vi "ProScan 3 Stage Engine.vi"(0 "Pro Scan 3 Notifier Name":string="ProScan3", 11 "COM Port":string[](array[string])) -> ()   [LabVIEW 2016]
uses:
  Stages Controls/Stage Notifier Element.ctl
  Stages Controls/Stage Actions.ctl
  Stages Controls/Stage Status.ctl
  <vilib>/Instr/_visa.llb/VISA Configure Serial Port (Instr).vi
panel:
  out "Backlash Status":string
  in  "Get Position":bool
  in  "XY Step Size (µm)":dbl format="%#_4g"
  in  "Y Position (µm)":dbl format="%#_4g"
  in  "X Position (µm)":dbl format="%#_4g"
  in  "Home":bool
  in  "Right":bool
  in  "Left":bool
  in  "Down":bool
  in  "Halt":bool
  in  "Up":bool
  in  "Quit":bool
  # "NOTE: Positions do not live update."
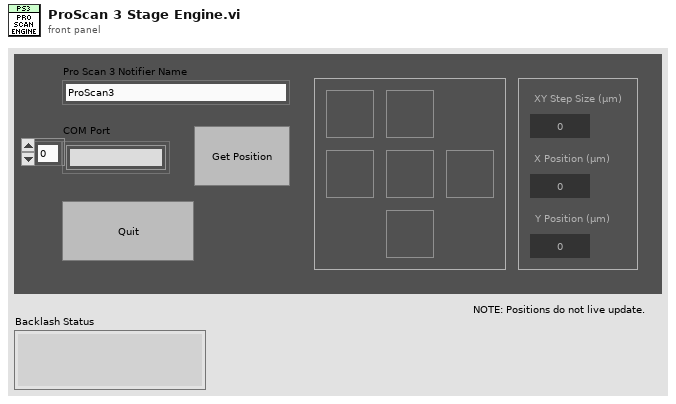
[diagram p1: front panel]
types:
  T1 = typedef "Stage Notifier Element.ctl" = cluster{"Action":T2, "Axis":bool[], "Setpoint":dbl[], "Velocity":dbl, "Cmd Recvd?":bool, "Position":dbl[], "Status":T3, "Misc":variant}
  T2 = typedef "Stage Actions.ctl" = enum16{"Get Position", "MVR", "MOVE", "HALT", "ONTARGET", "ERROR", "REFERENCE", "INIT", "VELOCITY", "STATUS", "EXIT", "HOME", "ZEROPOS", "NANOPOS", "ANALOG", "QUIT"}
  T3 = typedef "Stage Status.ctl" = enum16{"Error", "Abort", "Busy", "On Target"}
  T4 = enum32{"Invalid", "Standard", "Closed", "Hidden", "Minimized", "Maximized"}
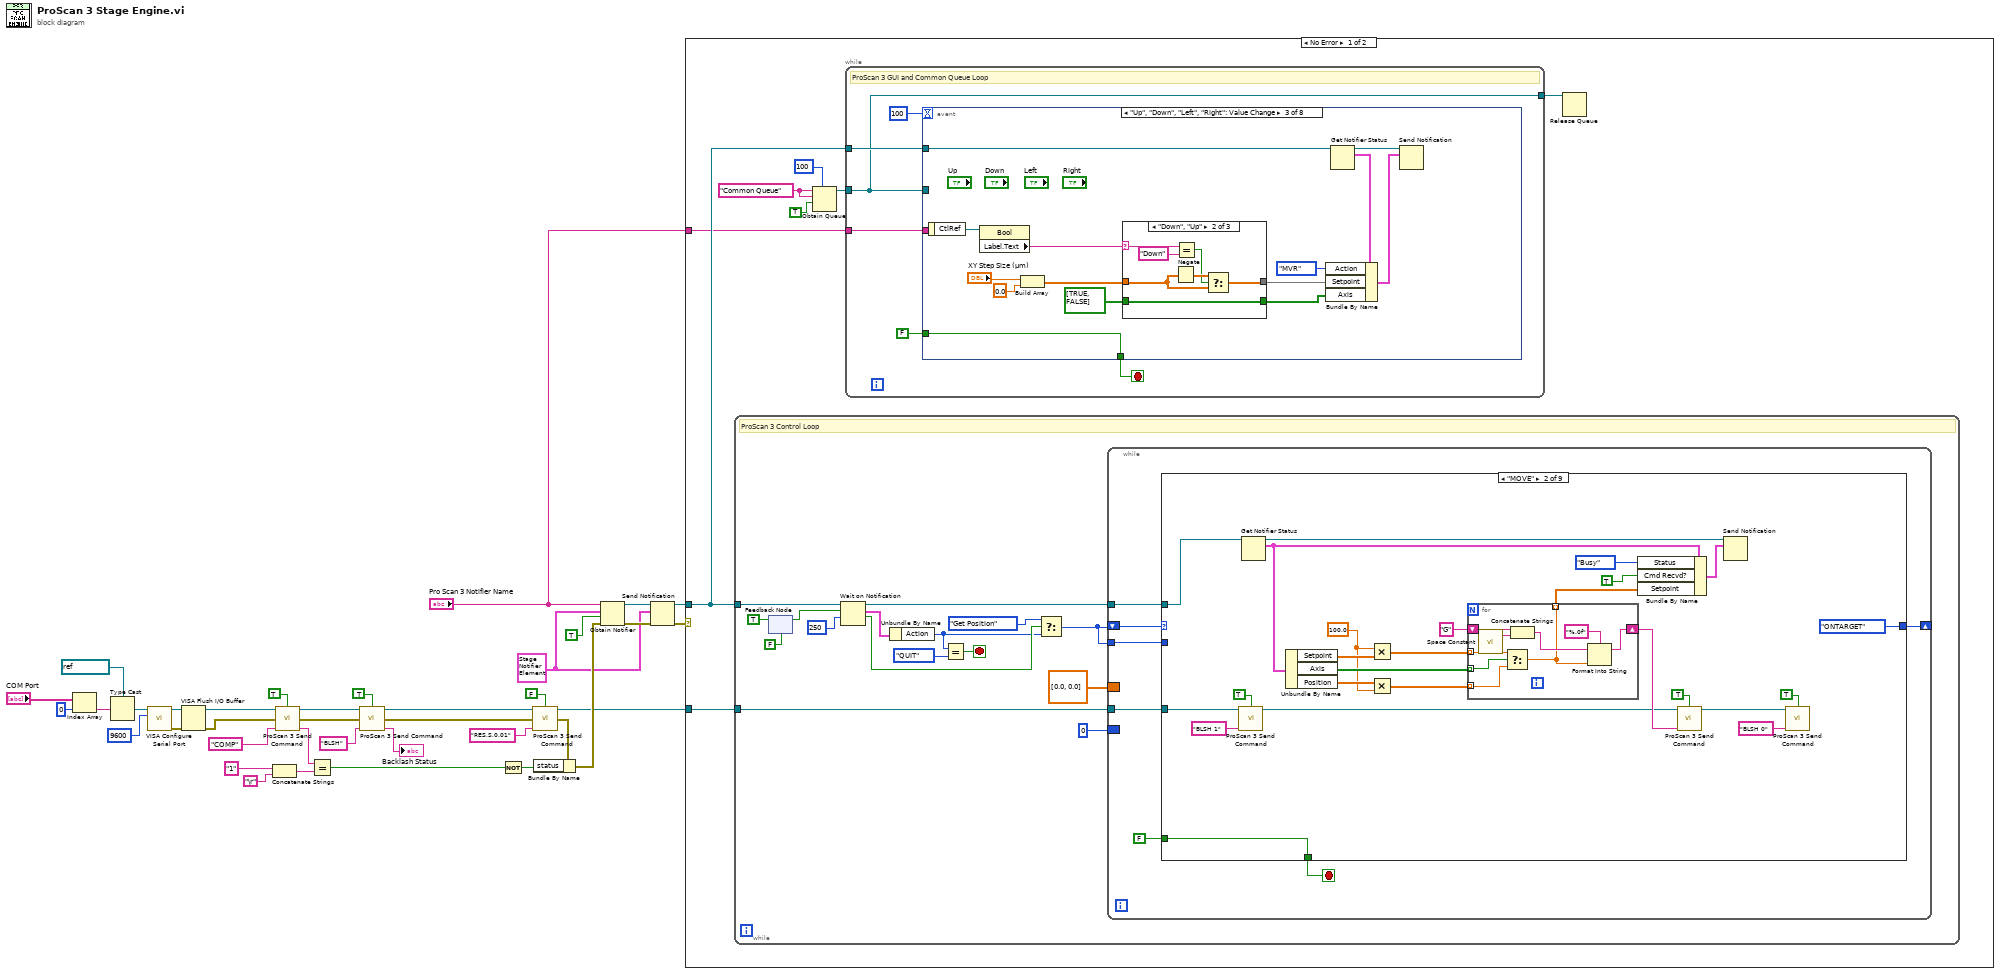
[diagram p0: block diagram]
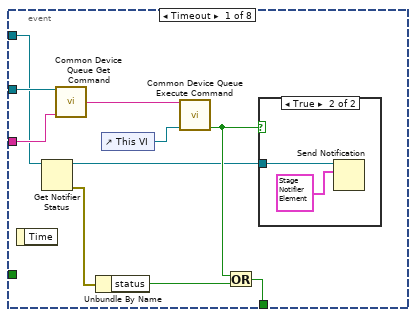
[diagram p2: hidden frame]
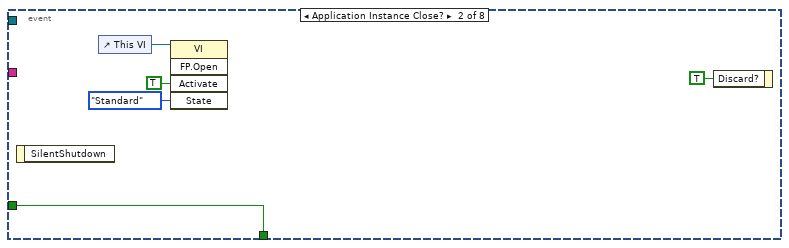
[diagram p4: hidden frame]
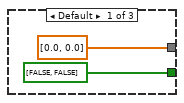
[diagram p5: hidden frame]
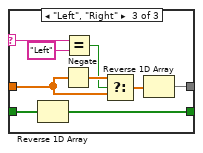
[diagram p6: hidden frame]
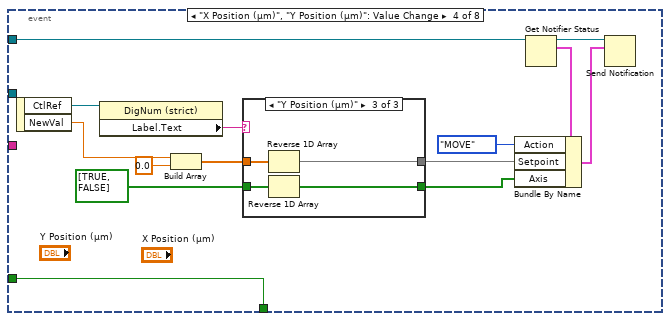
[diagram p7: hidden frame]
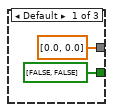
[diagram p8: hidden frame]
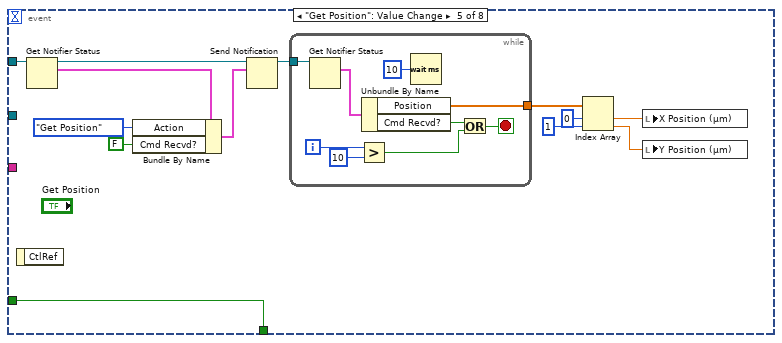
[diagram p10: hidden frame]
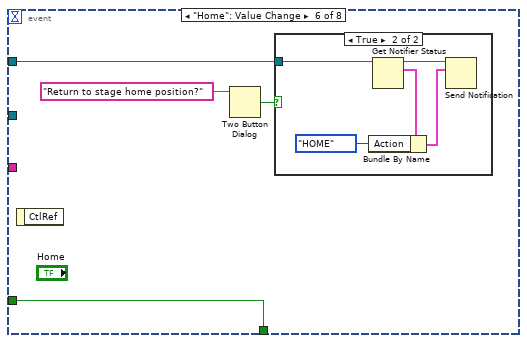
[diagram p11: hidden frame]
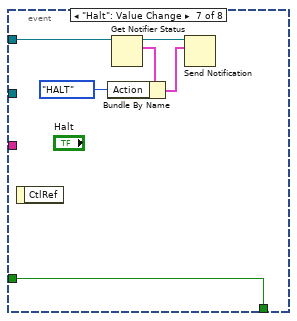
[diagram p13: hidden frame]
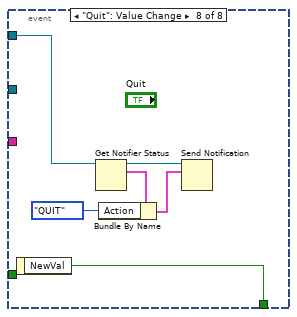
[diagram p14: hidden frame]
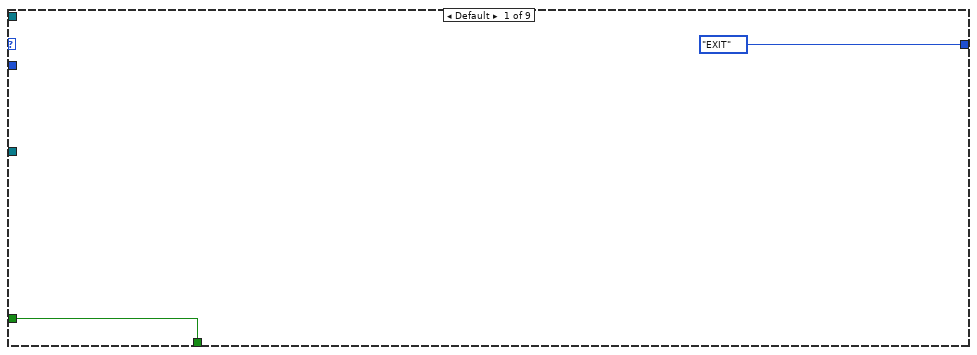
[diagram p15: hidden frame]
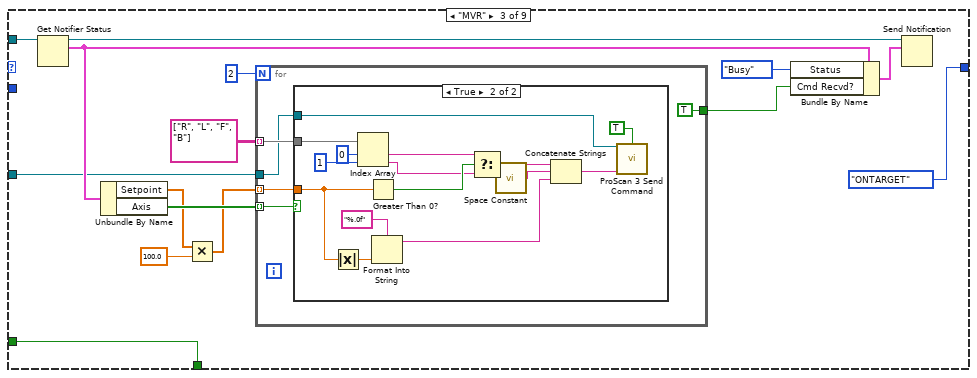
[diagram p16: hidden frame]
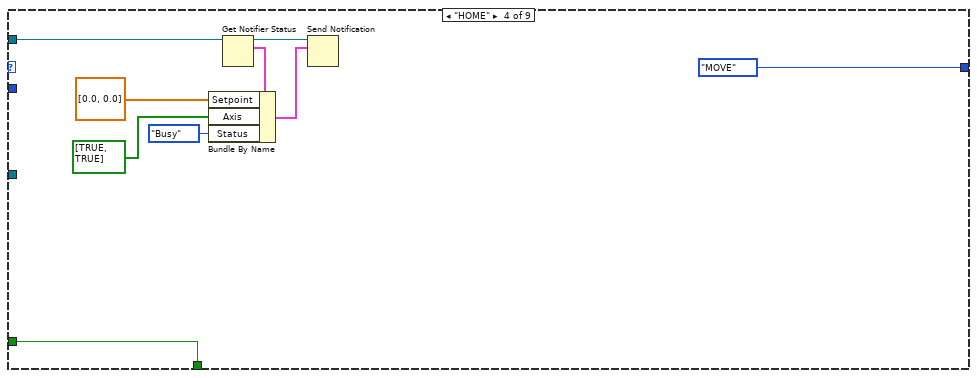
[diagram p18: hidden frame]
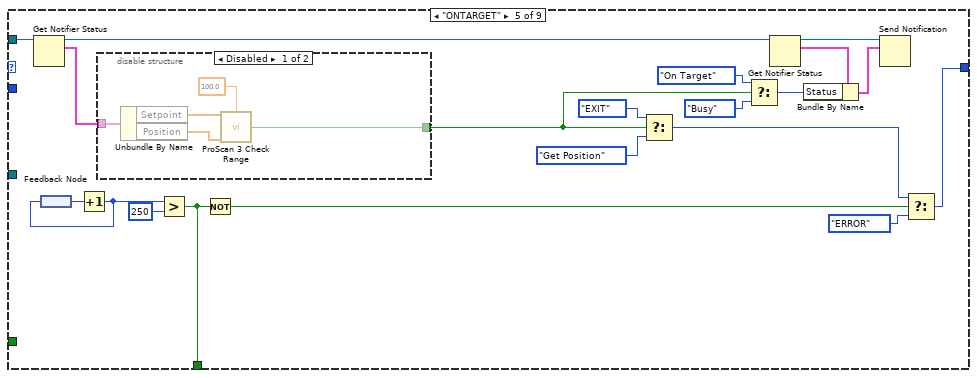
[diagram p19: hidden frame]
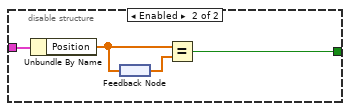
[diagram p20: hidden frame]
diagram:
  w19 = T1 {"Action"=enum."Get Position", "Axis"=[], "Setpoint"=[], "Velocity"=0.5, "Cmd Recvd?"=FALSE, "Position"=[], "Status"=enum."On Target", "Misc"=variant} ("Stage Status")
  n1 = Index Array(array="COM Port", index=0) -> (element=w15:string)
  n2 = Type Cast(type=refnum<visa-resource-name> "COM5" ("VISA resource name"), x=w15) -> (*(type *) &x=w14:refnum<visa-resource-name>)
  n3 = call-poly "VISA Configure Serial Port"("VISA resource name"=w14, "baud rate (9600)"=u32 9600) -> ("VISA resource name out"=w35:refnum<visa-resource-name>, "error out"=w34:errorcluster)  [unwired: 12 in]
  n4 = VISA Flush I/O Buffer(VISA resource name=w35, error in (no error)=w34) -> (VISA resource name out=w28:refnum<visa-resource-name>, error out=w27:errorcluster)  [unwired: 1 in]
  n5 = Concatenate Strings("1", "\r") -> (w31:string)
  n6 = call "ProScan 3 Send Command.vi"("VISA Ref"=w28, "Wait for Reply?"=TRUE, "Error In"=w27, "Command"="COMP") -> ("VISA Ref Out"=w5:refnum<visa-resource-name>, "Error Out"=w3:errorcluster, "Response"=w25:string)  [unwired: 9 in]
  n7 = Equal?(x=w25, y=w31) -> (x = y?=w30:bool)
  n8 = call "ProScan 3 Send Command.vi"("VISA Ref"=w5, "Wait for Reply?"=TRUE, "Error In"=w3, "Command"="BLSH") -> ("VISA Ref Out"=w4:refnum<visa-resource-name>, "Error Out"=w2:errorcluster, "Response"=→"Backlash Status":string)  [unwired: 9 in]
  n9 = Not(x=w30) -> (.not. x?=w29:bool)
  n10 = call "ProScan 3 Send Command.vi"("VISA Ref"=w4, "Wait for Reply?"=FALSE, "Error In"=w2, "Command"="RES,S,0.01") -> ("VISA Ref Out"=w11:refnum<visa-resource-name>, "Error Out"=w10:errorcluster)  [unwired: 9 in, 1 out]
  n11 = Bundle By Name(cluster=w10, "status"=w29) -> (w36:errorcluster)
  n12 = Obtain Notifier(name (unnamed)="Pro Scan 3 Notifier Name", notification data type=w19, create if not found? (T)=TRUE, error in (no error)=w36) -> (notifier out=w23:refnum<notifier>, error out=w22:errorcluster)  [unwired: 1 out]
  n13 = Send Notification(notification=w19, notifier=w23, error in (no error)=w22) -> (notifier out=w20:refnum<notifier>, error out=w21:errorcluster)
  n14 = case shown="No Error" w21 {
    selector: w21 -> [_ w408]
    tunnel: w20 -> [w41 w409]
    tunnel: w11 -> [w45 w410]
    tunnel: "Pro Scan 3 Notifier Name" -> [w40 _]
    frame No Error {
      w44 = "Common Queue" ("Unique Notifier Name")
      n15 = while {
        tunnel: w41 -> [w181]
        tunnel: w45 -> [w178]
        stop <- w177 stop-if-true
        # "ProScan 3 Control Loop"
        n16 = feedback-in #1(TRUE ("ignore previous (F)")) -> ()
        n17 = feedback #1(FALSE ("ignore previous (F)")) -> (w172:bool)
        n18 = Wait on Notification(notifier=w181, ignore previous (F)=w172, timeout in ms (-1)=250) -> (notifier out=w180:refnum<notifier>, notification=w176:T1, timed out?=w169:bool)  [unwired: 1 in, 1 out]
        n19 = Unbundle By Name(w176) -> ("Action"=w167:T2)
        n20 = Equal?(x=w167, y=Stage_Actions."QUIT") -> (x = y?=w177:bool)
        n21 = Select(t=Stage_Actions."Get Position", s=w169, f=w167) -> (s? t:f=w166:T2)
        n22 = while {
          tunnel: w180 -> [w188]
          tunnel: w178 -> [w186]
          shift-right: [w185] -> _
          shift-left: w166 -> [w187]
          tunnel: w166 -> [w182]
          border: 0 -> [_]
          border: dbl[] [0.0, 0.0] -> [_]
          stop <- w183 stop-if-true
          n23 = case shown="\"MOVE\"" w187 {
            selector: w187 -> [_ _ _ _ _ _ _ w362 _]
            tunnel: w188 -> [_ w211 w234 w264 w281 w319 w345 w364 w401]
            tunnel: w186 -> [_ w196 w229 _ _ w302 w350 w357 w399]
            tunnel: [Stage_Actions."EXIT" ("y") Stage_Actions."ONTARGET" ("y") Stage_Actions."ONTARGET" ("y") Stage_Actions."MOVE" ("y") w272 w304 w342 Stage_Actions."EXIT" ("y") Stage_Actions."QUIT" ("y")] -> w185
            tunnel: FALSE -> [w190 w215 w239 w262 _ w321 w338 _ _]
            tunnel: [w190 w215 w239 w262 w275 w321 w338 TRUE TRUE] -> w183
            tunnel: w182 -> [_ _ _ _ _ w303 _ _ _]
            frame Default {
            }
            frame "MOVE" {
              w200 = 100.0
              n24 = call "ProScan 3 Send Command.vi"("VISA Ref"=w196, "Wait for Reply?"=TRUE, "Command"="BLSH 1") -> ("VISA Ref Out"=w195:refnum<visa-resource-name>)  [unwired: 10 in, 2 out]
              n25 = Get Notifier Status(notifier=w211) -> (notifier out=w213:refnum<notifier>, current notification=w206:T1)  [unwired: 1 in, 3 out]
              n26 = Unbundle By Name(w206) -> ("Setpoint"=w202:dbl[], "Axis"=w207:bool[], "Position"=w201:dbl[])
              n27 = Multiply(x=w200, y=w202) -> (x*y=w198:dbl[])
              n28 = Multiply(x=w201, y=w200) -> (x*y=w199:dbl[])
              n29 = for {
                tunnel: w207 -> [w223] mode=indexing
                tunnel: w199 -> [w217] mode=indexing
                tunnel: w198 -> [w224] mode=indexing
                shift-right: [w218] -> w203
                shift-left: "G" ("f") -> [w221]
                tunnel: [w216] -> w204 mode=indexing
                n30 = call <vilib>:"Space Constant.vi"() -> ("String"=w220:string)
                n31 = Select(t=w224, s=w223, f=w217) -> (s? t:f=w216:dbl)
                n32 = Concatenate Strings(w221, w220) -> (w219:string)
                n33 = Format Into String(format string="%.0f", initial string=w219, w216) -> (resulting string=w218:string)  [unwired: 1 in, 1 out]
              }
              n34 = Bundle By Name(cluster=w206, "Status"=Stage_Status."Busy", "Cmd Recvd?"=TRUE, "Setpoint"=w204) -> (w212:T1)
              n35 = call "ProScan 3 Send Command.vi"("VISA Ref"=w195, "Wait for Reply?"=TRUE, "Command"=w203) -> ("VISA Ref Out"=w191:refnum<visa-resource-name>)  [unwired: 10 in, 2 out]
              n36 = Send Notification(notification=w212, notifier=w213) -> ()  [unwired: 1 in, 2 out]
              n37 = call "ProScan 3 Send Command.vi"("VISA Ref"=w191, "Wait for Reply?"=TRUE, "Command"="BLSH 0") -> ()  [unwired: 10 in, 3 out]
            }
            frame "MVR" {
              n38 = Get Notifier Status(notifier=w234) -> (notifier out=w236:refnum<notifier>, current notification=w233:T1)  [unwired: 1 in, 3 out]
              n39 = Unbundle By Name(w233) -> ("Setpoint"=w227:dbl[], "Axis"=w232:bool[])
              n40 = Multiply(x=w227, y=100.0) -> (x*y=w225:dbl[])
              n41 = for {
                N: 2 -> [_]
                tunnel: w232 -> [w244] mode=indexing
                tunnel: w225 -> [w243] mode=indexing
                tunnel: string[][] [["R", "L"], ["F", "B"]] -> [w242] mode=indexing
                tunnel: w229 -> [w241]
                tunnel: [TRUE ("Cmd Recvd?")] -> w228
                n42 = case shown="True" w244 {
                  tunnel: w243 -> [_ w252]
                  tunnel: w242 -> [_ w259]
                  tunnel: w241 -> [_ w245]
                  frame False {
                  }
                  frame True {
                    n43 = Absolute Value(x=w252) -> (abs(x)=w248:dbl)
                    n44 = Index Array(array=w259, index #1=0 ("index"), index #2=1 ("index")) -> (element #1=w254:string, element #2=w255:string)
                    n45 = Greater Than 0?(x=w252) -> (x > 0?=w256:bool)
                    n46 = Format Into String(format string="%.0f", w248) -> (resulting string=w249:string)  [unwired: 2 in, 1 out]
                    n47 = Select(t=w254, s=w256, f=w255) -> (s? t:f=w251:string)
                    n48 = call <vilib>:"Space Constant.vi"() -> ("String"=w250:string)
                    n49 = Concatenate Strings(w251, w250, w249) -> (w246:string)
                    n50 = call "ProScan 3 Send Command.vi"("VISA Ref"=w245, "Wait for Reply?"=TRUE, "Command"=w246) -> ()  [unwired: 10 in, 3 out]
                  }
                }
              }
              n51 = Bundle By Name(cluster=w233, "Status"=Stage_Status."Busy", "Cmd Recvd?"=w228) -> (w235:T1)
              n52 = Send Notification(notification=w235, notifier=w236) -> ()  [unwired: 1 in, 2 out]
            }
            frame "HOME" {
              n53 = Get Notifier Status(notifier=w264) -> (notifier out=w266:refnum<notifier>, current notification=w267:T1)  [unwired: 1 in, 3 out]
              n54 = Bundle By Name(cluster=w267, "Setpoint"=dbl[] [0.0, 0.0], "Axis"=bool[] [TRUE, TRUE], "Status"=Stage_Status."Busy") -> (w265:T1)
              n55 = Send Notification(notification=w265, notifier=w266) -> ()  [unwired: 1 in, 2 out]
            }
            frame "ONTARGET" {
              n56 = Get Notifier Status(notifier=w281) -> (notifier out=w280:refnum<notifier>, current notification=w279:T1)  [unwired: 1 in, 3 out]
              n57 = feedback #2() -> (w278:i32)
              n58 = Increment(x=w278) -> (x+1=w277:i32)
              n59 = feedback-in #2(w277) -> ()
              n60 = disable-structure shown="Disabled" {
                disable-tunnel: w279 -> [w293 w297]
                disable-tunnel: [w289 w294] -> w269
                frame Disabled {
                  n61 = Unbundle By Name(w293) -> ("Setpoint"=w292:dbl[], "Position"=w291:dbl[])
                  n62 = call "ProScan 3 Check Range.vi"("Setpoint"=w292, "Range Limit"=100.0, "Position"=w291) -> ("In Range?"=w289:bool)  [unwired: 12 in]
                }
                frame Enabled {
                  n63 = Unbundle By Name(w297) -> ("Position"=w295:dbl[])
                  n64 = feedback-in #3(w295) -> ()
                  n65 = feedback #3() -> (w296:dbl[])
                  n66 = Equal?(x=w295, y=w296) -> (x = y?=w294:bool)
                }
              }
              n67 = Greater?(x=w277, y=250) -> (0:w275:bool)
              n68 = Not(x=w275) -> (.not. x?=w271:bool)
              n69 = Select(t=Stage_Actions."EXIT" ("y"), s=w269, f=Stage_Actions."Get Position" ("y")) -> (s? t:f=w274:T2)
              n70 = Select(t=Stage_Status."On Target" ("Status"), s=w269, f=Stage_Status."Busy" ("Status")) -> (s? t:f=w282:T3)
              n71 = Get Notifier Status(notifier=w280) -> (notifier out=w286:refnum<notifier>, current notification=w287:T1)  [unwired: 1 in, 3 out]
              n72 = Bundle By Name(cluster=w287, "Status"=w282) -> (w285:T1)
              n73 = Send Notification(notification=w285, notifier=w286) -> ()  [unwired: 1 in, 2 out]
              n74 = Select(t=w274, s=w271, f=Stage_Actions."ERROR") -> (s? t:f=w272:T2)
            }
            frame "Get Position" {
              w312 = "," ("regular expression")
              n75 = VISA Flush I/O Buffer(VISA resource name=w302) -> (VISA resource name out=w301:refnum<visa-resource-name>)  [unwired: 2 in, 1 out]
              n76 = call "ProScan 3 Send Command.vi"("VISA Ref"=w301, "Wait for Reply?"=TRUE, "Command"="P") -> ("Response"=w307:string)  [unwired: 10 in, 2 out]
              n77 = Search and Replace String(input string=w307, search string="[a-zA-Z]", replace string="") -> (result string=w310:string)  [unwired: 5 in, 3 out]
              n78 = Match Pattern(string=w310, regular expression=w312) -> (before substring=w313:string, after substring=w311:string)  [unwired: 1 in, 2 out]
              n79 = Match Pattern(string=w311, regular expression=w312) -> (before substring=w314:string, after substring=w315:string)  [unwired: 1 in, 2 out]
              n80 = Build Array(w313, w314, w315) -> (w316:string[])
              n81 = for {
                N: 2 -> [_]
                tunnel: w316 -> [w335] mode=indexing
                tunnel: [w333] -> w300 mode=indexing
                n82 = call <vilib>:"Trim Whitespace.vi"("string"=w335) -> ("trimmed string"=w332:string)  [unwired: 1 in]
                n83 = Decimal String To Number(string=w332, default (0L)=0.0) -> (number=w333:dbl)  [unwired: 1 in, 1 out]
              }
              n84 = Divide(x=w300, y=100.0) -> (x/y=w298:dbl[])
              n85 = Get Notifier Status(notifier=w319) -> (notifier out=w322:refnum<notifier>, current notification=w306:T1)  [unwired: 1 in, 3 out]
              n86 = case shown="Default" w303 {
                tunnel: w306 -> [w326 w331]
                tunnel: [w325 w330] -> w305
                tunnel: w298 -> [w324 w329]
                tunnel: [Stage_Actions."ONTARGET" ("y") Stage_Actions."EXIT" ("y")] -> w304
                frame Default {
                  n87 = Bundle By Name(cluster=w326, "Position"=w324) -> (w325:T1)
                }
                frame "Get Position", "HALT" {
                  n88 = Bundle By Name(cluster=w331, "Position"=w329, "Cmd Recvd?"=TRUE) -> (w330:T1)
                }
              }
              n89 = Send Notification(notification=w305, notifier=w322) -> ()  [unwired: 1 in, 2 out]
            }
            frame "HALT" {
              n90 = call "ProScan 3 Send Command.vi"("VISA Ref"=w350, "Wait for Reply?"=TRUE, "Command"="I" ("string")) -> ("Response"=w351:string)  [unwired: 10 in, 2 out]
              n91 = Concatenate Strings("R" ("y"), "\r") -> (w353:string)
              n92 = Equal?(x=w351, y=w353) -> (x = y?=w341:bool)
              n93 = Select(t=Stage_Status."Abort" ("Status"), s=w341, f=Stage_Status."Error" ("Status")) -> (s? t:f=w337:T3)
              n94 = Select(t=Stage_Actions."Get Position" ("y"), s=w341, f=Stage_Actions."ERROR" ("y")) -> (s? t:f=w342:T2)
              n95 = Get Notifier Status(notifier=w345) -> (notifier out=w348:refnum<notifier>, current notification=w349:T1)  [unwired: 1 in, 3 out]
              n96 = Bundle By Name(cluster=w349, "Status"=w337, "Cmd Recvd?"=TRUE) -> (w347:T1)
              n97 = Send Notification(notification=w347, notifier=w348) -> ()  [unwired: 1 in, 2 out]
            }
            frame "ERROR".."EXIT" {
              n98 = case shown="Default" w362 {
                tunnel: w364 -> [w390 w396]
                tunnel: [w390 w391] -> w356
                frame Default {
                }
                frame "ERROR" {
                  n99 = Get Notifier Status(notifier=w396) -> (notifier out=w393:refnum<notifier>, current notification=w395:T1)  [unwired: 1 in, 3 out]
                  n100 = Bundle By Name(cluster=w395, "Status"=Stage_Status."Error") -> (w392:T1)
                  n101 = Send Notification(notification=w392, notifier=w393) -> (notifier out=w391:refnum<notifier>)  [unwired: 1 in, 1 out]
                }
              }
              n102 = Get Notifier Status(notifier=w356) -> (notifier out=w360:refnum<notifier>, current notification=w359:T1)  [unwired: 1 in, 3 out]
              n103 = disable-structure shown="Enabled" {
                disable-tunnel: w359 -> [w371 w389]
                disable-tunnel: [w370 w389] -> w358
                disable-tunnel: w357 -> [w365 _]
                frame Disabled {
                  w377 = "," ("regular expression")
                  n104 = VISA Flush I/O Buffer(VISA resource name=w365) -> (VISA resource name out=w369:refnum<visa-resource-name>)  [unwired: 2 in, 1 out]
                  n105 = call "ProScan 3 Send Command.vi"("VISA Ref"=w369, "Wait for Reply?"=TRUE, "Command"="P") -> ("Response"=w372:string)  [unwired: 10 in, 2 out]
                  n106 = Search and Replace String(input string=w372, search string="[a-zA-Z]", replace string="") -> (result string=w375:string)  [unwired: 5 in, 3 out]
                  n107 = Match Pattern(string=w375, regular expression=w377) -> (before substring=w378:string, after substring=w376:string)  [unwired: 1 in, 2 out]
                  n108 = Match Pattern(string=w376, regular expression=w377) -> (before substring=w379:string, after substring=w380:string)  [unwired: 1 in, 2 out]
                  n109 = Build Array(w378, w379, w380) -> (w381:string[])
                  n110 = for {
                    N: 2 -> [_]
                    tunnel: w381 -> [w388] mode=indexing
                    tunnel: [w386] -> w368 mode=indexing
                    n111 = call <vilib>:"Trim Whitespace.vi"("string"=w388) -> ("trimmed string"=w385:string)  [unwired: 1 in]
                    n112 = Decimal String To Number(string=w385, default (0L)=0.0) -> (number=w386:dbl)  [unwired: 1 in, 1 out]
                  }
                  n113 = Divide(x=w368, y=100.0) -> (x/y=w366:dbl[])
                  n114 = Bundle By Name(cluster=w371, "Position"=w366) -> (w370:T1)
                }
                frame Enabled {
                }
              }
              n115 = Send Notification(notification=w358, notifier=w360) -> ()  [unwired: 1 in, 2 out]
            }
            frame "QUIT" {
              n116 = Release Notifier(notifier=w401, force destroy? (F)=TRUE) -> ()  [unwired: 1 in, 3 out]
              n117 = VISA Close(VISA resource name=w399) -> ()  [unwired: 1 in, 1 out]
            }
          }
        }
      }
      n118 = Obtain Queue(max queue size (-1, unlimited)=100, name (unnamed)=w44, element data type=w44, create if not found? (T)=TRUE) -> (queue out=w42:refnum<queue>)  [unwired: 1 in, 2 out]
      n119 = while {
        tunnel: w42 -> [w46]
        tunnel: w40 -> [w49]
        tunnel: w41 -> [w50]
        tunnel: [w46] -> w38
        stop <- w48 stop-if-true
        # "ProScan 3 GUI and Common Queue Loop"
        n120 = event shown="[2] \"Up\", \"Down\", \"Left\", \"Right\": Value Change" {
          selector: _ -> [_ _ _ _ _ _ _ _]
          dyn-events: _ -> [_ _ _ _ _ _ _ _]
          timeout: 100 -> [_ _ _ _ _ _ _ _]
          tunnel: w46 -> [w55 _ _ _ _ _ _ _]
          tunnel: w50 -> [w52 _ w75 w107 w134 w145 w158 w165]
          tunnel: w49 -> [w54 _ _ _ _ _ _ _]
          tunnel: [w53 w68 w78 w114 w135 w147 w159 w161] -> w48
          tunnel: FALSE -> [_ w68 w78 w114 w135 w147 w159 _]
          event Timeout {
            n121 = event-data() -> ()  [unwired: 1 in, 1 out]
            n122 = Get Notifier Status(notifier=w52) -> (notifier out=w56:refnum<notifier>, error out=w61:errorcluster)  [unwired: 1 in, 3 out]
            n123 = call "Common Device Queue Get Command.vi"("Common Queue"=w55, "Notifier Name"=w54) -> ("Command"=w60:string)  [unwired: 12 in, 1 out]
            n124 = Unbundle By Name(w61) -> ("status"=w58:bool)
            n125 = control-ref of="This VI"() -> (w59:refnum<vi>)
            n126 = call "Common Device Queue Execute Command.vi"("Common Command"=w60, "VI Refnum"=w59) -> ("Quit?"=w57:bool)  [unwired: 12 in, 1 out]
            n127 = Or(x=w57, y=w58) -> (x .or. y?=w53:bool)
            n128 = case shown="True" w57 {
              tunnel: w56 -> [_ w63]
              frame False {
              }
              frame True {
                n129 = Send Notification(notification=T1 {"Action"=enum."QUIT", "Axis"=[], "Setpoint"=[], "Velocity"=0.5, "Cmd Recvd?"=FALSE, "Position"=[], "Status"=enum."Error", "Misc"=variant} ("Stage Status"), notifier=w63) -> ()  [unwired: 1 in, 2 out]
              }
            }
          }
          event Application Instance Close? {
            n130 = event-data() -> ()  [unwired: 1 in, 1 out]
            n131 = control-ref of="This VI"() -> (w65:refnum<vi>)
            n132 = invoke class="VI" method="FP.Open"(reference=w65, "Activate"=TRUE ("Activate?"), "State"=T4."Standard") -> ()  [unwired: 2 in, 5 out]
            n133 = event-data("Discard?"=TRUE) -> ()  [unwired: 1 in, 1 out]
          }
          event "Up", "Down", "Left", "Right": Value Change {
            n134 = event-data() -> ("CtlRef"=w77:refnum<vi>)  [unwired: 1 in]
            n135 = property class="Bool"(reference=w77) -> ("Label.Text"=w82:string)  [unwired: 1 in, 2 out]
            n136 = Build Array("XY Step Size (µm)", 0.0 ("element")) -> (w80:dbl[])
            n137 = case shown="\"Down\", \"Up\"" w82 {
              selector: w82 -> [_ w91 w97]
              tunnel: w80 -> [_ w88 w96]
              tunnel: bool[] [TRUE, FALSE] -> [_ w85 w94]
              tunnel: [dbl[] [0.0, 0.0] w87 w93] -> w73
              tunnel: [bool[] [FALSE, FALSE] w85 w92] -> w72
              frame Default {
              }
              frame "Down", "Up" {
                n138 = Negate(x=w88) -> (-x=w89:dbl[])
                n139 = Equal?(x=w91, y="Down") -> (x = y?=w86:bool)
                n140 = Select(t=w89, s=w86, f=w88) -> (s? t:f=w87:dbl[])
              }
              frame "Left", "Right" {
                n141 = Reverse 1D Array(array=w94) -> (reversed array=w92:bool[])
                n142 = Negate(x=w96) -> (-x=w99:dbl[])
                n143 = Equal?(x=w97, y="Left") -> (x = y?=w98:bool)
                n144 = Select(t=w99, s=w98, f=w96) -> (s? t:f=w95:dbl[])
                n145 = Reverse 1D Array(array=w95) -> (reversed array=w93:dbl[])
              }
            }
            n146 = Get Notifier Status(notifier=w75) -> (notifier out=w70:refnum<notifier>, current notification=w74:T1)  [unwired: 1 in, 3 out]
            n147 = Bundle By Name(cluster=w74, "Action"=Stage_Actions."MVR", "Setpoint"=w73, "Axis"=w72) -> (w69:T1)
            n148 = Send Notification(notification=w69, notifier=w70) -> ()  [unwired: 1 in, 2 out]
          }
          event "X Position (µm)", "Y Position (µm)": Value Change {
            n149 = event-data() -> ("CtlRef"=w109:refnum<vi>, "NewVal"=w108:dbl)  [unwired: 1 in]
            n150 = property class="DigNum (strict)"(reference=w109) -> ("Label.Text"=w112:string)  [unwired: 1 in, 2 out]
            n151 = Build Array(w108, 0.0 ("element")) -> (w113:dbl[])
            n152 = case shown="\"Y Position (µm)\"" w112 {
              tunnel: w113 -> [_ w118 w122]
              tunnel: bool[] [TRUE, FALSE] -> [_ w117 w121]
              tunnel: [dbl[] [0.0, 0.0] w118 w120] -> w104
              tunnel: [bool[] [FALSE, FALSE] w117 w119] -> w103
              frame Default {
              }
              frame "X Position (µm)" {
              }
              frame "Y Position (µm)" {
                n153 = Reverse 1D Array(array=w122) -> (reversed array=w120:dbl[])
                n154 = Reverse 1D Array(array=w121) -> (reversed array=w119:bool[])
              }
            }
            n155 = Get Notifier Status(notifier=w107) -> (notifier out=w106:refnum<notifier>, current notification=w105:T1)  [unwired: 1 in, 3 out]
            n156 = Bundle By Name(cluster=w105, "Action"=Stage_Actions."MOVE", "Setpoint"=w104, "Axis"=w103) -> (w101:T1)
            n157 = Send Notification(notification=w101, notifier=w106) -> ()  [unwired: 1 in, 2 out]
          }
          event "Get Position": Value Change {
            n158 = event-data() -> ()  [unwired: 1 in, 1 out]
            n159 = Get Notifier Status(notifier=w134) -> (notifier out=w133:refnum<notifier>, current notification=w132:T1)  [unwired: 1 in, 3 out]
            n160 = Bundle By Name(cluster=w132, "Action"=Stage_Actions."Get Position", "Cmd Recvd?"=FALSE) -> (w129:T1)
            n161 = Send Notification(notification=w129, notifier=w133) -> (notifier out=w128:refnum<notifier>)  [unwired: 1 in, 1 out]
            n162 = while {
              tunnel: w128 -> [w144]
              tunnel: [w136] -> w127
              i -> [w140]
              stop <- w137 stop-if-true
              n163 = Get Notifier Status(notifier=w144) -> (current notification=w143:T1)  [unwired: 1 in, 4 out]
              n164 = Greater?(x=w140, y=10) -> (0:w138:bool)
              n165 = Unbundle By Name(w143) -> ("Position"=w136:dbl[], "Cmd Recvd?"=w139:bool)
              n166 = Wait (ms)(milliseconds to wait=u32 10) -> ()  [unwired: 1 out]
              n167 = Or(x=w139, y=w138) -> (x .or. y?=w137:bool)
            }
            n168 = Index Array(array=w127, index #1=0 ("index"), index #2=1 ("index")) -> (element #1=w124:dbl, element #2=w123:dbl)
            n169 = local write "X Position (µm)"(w124) -> ()
            n170 = local write "Y Position (µm)"(w123) -> ()
          }
          event "Home": Value Change {
            n171 = event-data() -> ()  [unwired: 1 in, 1 out]
            n172 = Two Button Dialog(message="Return to stage home position?") -> (T button?=w146:bool)  [unwired: 2 in]
            n173 = case shown="True" w146 {
              tunnel: w145 -> [_ w153]
              frame False {
              }
              frame True {
                n174 = Get Notifier Status(notifier=w153) -> (notifier out=w152:refnum<notifier>, current notification=w151:T1)  [unwired: 1 in, 3 out]
                n175 = Bundle By Name(cluster=w151, "Action"=Stage_Actions."HOME") -> (w150:T1)
                n176 = Send Notification(notification=w150, notifier=w152) -> ()  [unwired: 1 in, 2 out]
              }
            }
          }
          event "Halt": Value Change {
            n177 = event-data() -> ()  [unwired: 1 in, 1 out]
            n178 = Get Notifier Status(notifier=w158) -> (notifier out=w157:refnum<notifier>, current notification=w156:T1)  [unwired: 1 in, 3 out]
            n179 = Bundle By Name(cluster=w156, "Action"=Stage_Actions."HALT") -> (w155:T1)
            n180 = Send Notification(notification=w155, notifier=w157) -> ()  [unwired: 1 in, 2 out]
          }
          event "Quit": Value Change {
            n181 = event-data() -> ("NewVal"=w161:bool)  [unwired: 1 in]
            n182 = Get Notifier Status(notifier=w165) -> (notifier out=w164:refnum<notifier>, current notification=w163:T1)  [unwired: 1 in, 3 out]
            n183 = Bundle By Name(cluster=w163, "Action"=Stage_Actions."QUIT") -> (w162:T1)
            n184 = Send Notification(notification=w162, notifier=w164) -> ()  [unwired: 1 in, 2 out]
          }
        }
      }
      n185 = Release Queue(queue=w38) -> ()  [unwired: 2 in, 3 out]
    }
    frame Error {
      n186 = VISA Close(VISA resource name=w410) -> ()  [unwired: 1 in, 1 out]
      n187 = Release Notifier(notifier=w409, force destroy? (F)=TRUE, error in (no error)=w408) -> (error out=w406:errorcluster)  [unwired: 2 out]
      n188 = Unbundle By Name(w406) -> ("source"=w403:string)
      n189 = Concatenate Strings("Pro Scan 3 Error", "\r", w403) -> (w402:string)
      n190 = One Button Dialog(message=w402) -> ()  [unwired: 1 in, 1 out]
    }
  }
